vi "Utility.RestartTarget.vi"(8 "error in (no error)":errorcluster, 11 "Target (localhost)":refnum<k21>="localhost") -> (0 "error out":errorcluster)   [LabVIEW 2014, in "ParametericRoutines.lvlib"]
uses:
  ParametericRoutines.lvlib
  <vilib>/nisyscfg/Close (System).vi
  <vilib>/nisyscfg/nisyscfg.lvlib
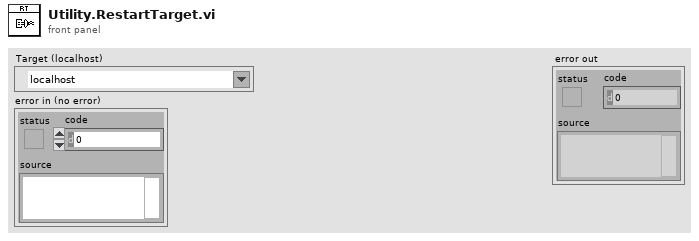
[diagram p1: front panel]
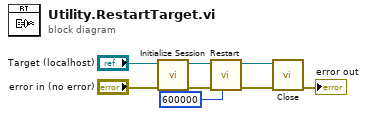
[diagram p0: block diagram]
diagram:
  n1 = call <vilib>:"Initialize Session.vi"("error in (no error)"="error in (no error)", "Target (localhost)"="Target (localhost)") -> ("error out"=w7:errorcluster, "Session out"=w6:refnum<k21>)  [unwired: 8 in]
  n2 = call <vilib>:"Restart.vi"("Timeout (180,000 ms)"=u32 600000, "error in (no error)"=w7, "Session in"=w6) -> ("error out"=w5:errorcluster, "Session out"=w4:refnum<k21>)  [unwired: 6 in, 1 out]
  n3 = call-poly <vilib>:"Close.vi"("error in (no error)"=w5, "Session in"=w4) -> ("error out"=→"error out":errorcluster)  [unwired: 9 in]
